vi "StreamReceiveAcquisitionChA.vi"() -> ()   [LabVIEW 2018]
uses:
  <resource>/objmgr/ni.dex.rc
panel:
  in  "stop":bool
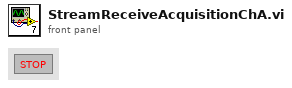
[diagram p1: front panel]
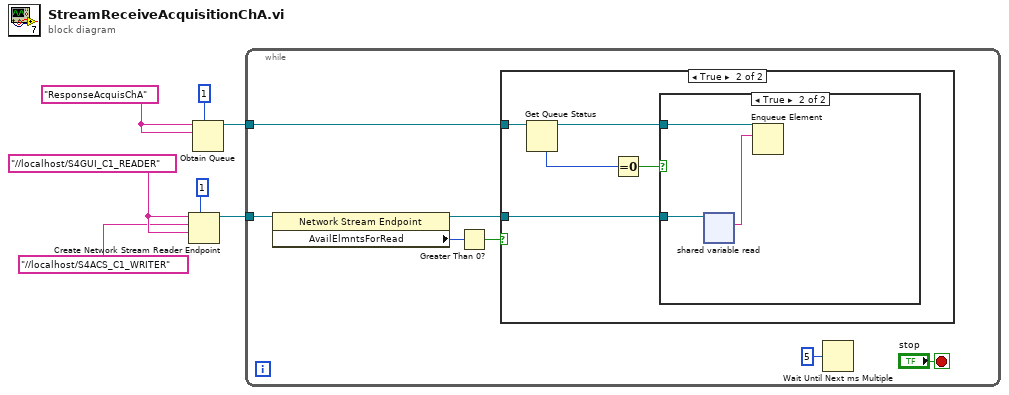
[diagram p0: block diagram]
diagram:
  w2 = "//localhost/S4GUI_C1_READER"
  w7 = "ResponseAcquisChA"
  n1 = Create Network Stream Reader Endpoint(7:1 ("reader buffer size"), 9:w2, 10:"//localhost/S4ACS_C1_WRITER", 11:w2) -> (3:w4:refnum<k21>)  [unwired: 3 in, 1 out]
  n2 = Obtain Queue(max queue size (-1, unlimited)=1, name (unnamed)=w7, element data type=w7) -> (queue out=w6:refnum<queue>)  [unwired: 2 in, 2 out]
  n3 = while {
    tunnel: w6 -> [w13]
    tunnel: w4 -> [w12]
    stop <- "stop" stop-if-true
    n4 = property class="Network Stream Endpoint"(reference=w12) -> (reference out=w11:refnum<k21>, "AvailElmntsForRead"=w10:i32)  [unwired: 1 in, 1 out]
    n5 = Greater Than 0?(x=w10) -> (x > 0?=w9:bool)
    n6 = case shown="True" w9 {
      tunnel: w13 -> [_ w16]
      tunnel: w11 -> [_ w19]
      frame False {
      }
      frame True {
        n7 = Get Queue Status(queue=w16) -> (queue out=w15:refnum<queue>, # elements in queue=w18:i32)  [unwired: 2 in, 6 out]
        n8 = Equal To 0?(x=w18) -> (x = 0?=w17:bool)
        n9 = case shown="True" w17 {
          tunnel: w19 -> [_ w22]
          tunnel: w15 -> [_ w20]
          frame False {
          }
          frame True {
            n10 = shared-variable-read(w22) -> (w21:string)  [unwired: 2 in, 3 out]
            n11 = Enqueue Element(queue=w20, element=w21) -> ()  [unwired: 2 in, 3 out]
          }
        }
      }
    }
    n12 = Wait Until Next ms Multiple(millisecond multiple=u32 5) -> ()  [unwired: 1 out]
  }
